vi "TDC_DAQV18_NewStructure.vi"(8 "error in (no error)":errorcluster, 9 "stop":bool, 10 "save data":bool, 11 "SMA mode":bool=TRUE) -> (3 "rate":dbl)   [LabVIEW 2017]
uses:
  <vilib>/Utility/file.llb/Write Delimited Spreadsheet (DBL).vi
  <vilib>/Utility/file.llb/Write Delimited Spreadsheet (I64).vi
panel:
  out "substring":string
  in  "factor":i32=128
  in  "displayCR":bool=TRUE
  in  "Counter Setting":dbl=100000.0 format="%#_13g"
  in  "replace dat":bool
  in  "append csv":bool=TRUE
  out "concatenated string":string
  out "number":u32=22
  out "element":string
  out "fine":u64=838 format="%x"
  in  "UDP Config":bool=TRUE
  in  "data  path":path=path "G:/tdc/2017"
  out "Array 6":u64[](array[numeric])
  out "cal 2":u64[](graph)
  in  "Thresholds (mV)":u16[](array[numeric])=[580, 580, 580, 580, 600, 600, 600, 600, 580, 580, 600, 600, 600, 600, 600, 600, 580, 580, 600, 600, 600, 600, 600, 600, 580, 580, 600, 600, 600, 600, 600, 600]
  out "error out 2":errorcluster={"status"=TRUE, "code"=1122, "source"="Dequeue Element in TDC_DAQV18_NewStructure.vi"}
  in  "display":bool=TRUE
  in  "Thresholds":u16=580
  in  "one key for threshold":bool=TRUE
  in  "RST":bool
  in  "通道数量":i32=64
  out "Cal Table":u32[](array[numeric])=[28636, 28570, 28472, 28284, 28524, 28354, 28408, 28049, 28174, 28071, 28126, 28086, 28151, 27908, 28025, 27898, 28233, 27859, 27914, 27888, 28140, 28038, 27911, 27738, 28022, 27827, 27982, 27675, 27862, 27768, 27841, 27799, 27874, 27627, 27754, 27650, 27959, 27594, 27633, 27606, 27668, 27555, 27455, 27220, 27394, 27187, 27334, 27119, 27301, 27220, 27267, 27235, 27336, 27057, 27150, 27031, 27376, 27049, 27063, 27028, 27283, 27180, 27100, 26881]
  in  "channel for cal":i32=62
  out "single":u32 format="%08x"
  out "channel number":u64
  in  "bytes to read":i32=320
  out "Calibration Counter":i32
  out "Event index":i32=97959
  out "cal":u32[](graph)=[0, 0, 0, 0, 0, 0, 0, 0, 0, 0, 0, 0, 0, 0, 0, 0, 0, 0, 0, 0, 0, 0, 0, 0, 0, 0, 0, 0, 0, 0, 0, 0, 0, 0, 0, 0, 0, 0, 0, 0, 0, 0, 0, 0, 0, 0, 0, 0, 0, 0, 0, 0, 0, 0, 0, 0, 0, 0, 0, 0, 0, 0, 0, 0, 0, 0, 0, 0, 0, 0, 0, 0, 0, 0, 0, 0, 0, 0, 0, 0, 0, 0, 0, 0, 0, 0, 0, 0, 0, 0, 0, 0, 0, 0, 0, 0, 0, 0, 0, 0, 0, 0, 0, 0, 0, 0, 0, 0, 0, 0, 0, 0, 0, 0, 0, 0, 0, 0, 0, 0, 0, 0, 0, 0, 0, 0, 0, 0, 0, 0, 0, 0, 0, 0, 0, 0, 0, 0, 0, 0, 0, 0, 0, 0, 0, 0, 0, 0, 0, 0, 0, 0, 0, 0, 0, 0, 0, 0, 0, 0, 0, 0, 0, 0, 0, 0, 0, 0, 0, 0, 0, 0, 0, 0, 0, 0, 0, 0, 0, 0, 0, 0, 0, 0, 0, 0, 0, 0, 0, 0, 0, 0, 0, 2, 54, 54, 14, 13, 87, 147, 41, 25, 155, 114, 17, 77, 15, 71, 56, 118, 81, 90, 49, 14, 113, 39, 20, 90, 64, 40, 165, 17, 96, 16, 10, 135, 156, 24, 21, 77, 15, 113, 60, 111, 60, 69, 56, 39, 25, 108, 23, 52, 40, 66, 77, 46, 18, 23, 25, 33, 46, 79, 55, 12, 43, 34, 54, 48, 32, 34, 28, 55, 22, 24, 21, 53, 50, 21, 11, 31, 77, 14, 70, 43, 17, 109, 25, 16, 16, 72, 32, 104, 58, 108, 13, 16, 11, 11, 72, 30, 49, 18, 45, 40, 66, 33, 22, 22, 74, 43, 18, 19, 21, 18, 60, 21, 31, 36, 29, 73, 97, 22, 11, 30, 9, 25, 193, 74, 57, 86, 69, 47, 59, 36, 30, 55, 41, 124, 44, 61, 22, 51, 50, 35, 27, 9, 64, 119, 23, 14, 164, 36, 42, 32, 43, 99, 31, 18, 26, 30, 31, 21, 113, 89, 30, 55, 19, 10, 21, 14, 46, 24, 51, 85, 44, 39, 50, 18, 26, 39, 30, 24, 32, 123, 21, 19, 90, 37, 44, 34, 33, 23, 68, 17, 29, 31, 65, 19, 61, 39, 31, 43, 29, 22, 10, 14, 11, 25, 86, 14, 22, 108, 89, 17, 47, 23, 15, 19, 146, 20, 31, 22, 74, 13, 22, 13, 120, 64, 70, 46, 27, 22, 133, 24, 44, 24, 20, 26, 110, 48, 68, 61, 65, 29, 49, 61, 92, 31, 33, 41, 54, 35, 24, 128, 22, 63, 41, 18, 84, 14, 25, 169, 23, 43, 15, 24, 172, 35, 124, 19, 31, 9, 11, 32, 134, 43, 65, 39, 44, 43, 34, 29, 13, 15, 74, 64, 26, 62, 44, 22, 21, 12, 14, 63, 43, 46, 39, 79, 28, 18, 24, 26, 73, 18, 22, 20, 21, 21, 45, 57, 75, 13, 62, 24, 20, 15, 60, 59, 77, 31, 32, 101, 20, 15, 29, 57, 76, 24, 48, 14, 20, 52, 70, 46, 31, 50, 8, 33, 45, 69, 28, 19, 14, 34, 17, 20, 68, 48, 88, 65, 48, 62, 27, 17, 28, 31, 70, 94, 13, 86, 14, 11, 31, 25, 51, 70, 22, 47, 24, 38, 30, 7, 11, 22, 25, 41, 15, 36, 52, 72, 54, 27, 28, 76, 34, 223, 31, 29, 41, 34, 92, 122, 60, 26, 43, 22, 56, 11, 24, 41, 50, 55, 18, 67, 41, 16, 30, 55, 27, 19, 61, 33, 85, 80, 79, 46, 14, 91, 48, 205, 23, 26, 18, 31, 58, 81, 35, 82, 83, 21, 37, 25, 26, 84, 60, 84, 13, 86, 69, 63, 74, 18, 117, 49, 45, 144, 12, 45, 13, 13, 74, 48, 19, 27, 51, 34, 25, 11, 11, 17, 100, 16, 10, 10, 59, 35, 84, 24, 26, 22, 20, 21, 11, 121, 83, 35, 36, 135, 15, 24, 41, 23, 27, 15, 35, 93, 35, 80, 24, 36, 29, 18, 16, 27, 17, 58, 12, 23, 32, 55, 89, 67, 14, 19, 26, 20, 122, 72, 55, 67, 25, 32, 18, 21, 46, 102, 133, 24, 22, 15, 47, 28, 29, 16, 17, 21, 26, 69, 27, 65, 58, 23, 21, 51, 56, 33, 62, 116, 37, 78, 49, 52, 75, 18, 48, 48, 16, 74, 24, 30, 58, 18, 32, 53, 19, 13, 9, 27, 13, 20, 38, 86, 118, 15, 12, 22, 31, 91, 25, 46, 133, 27, 15, 36, 45, 53, 133, 56, 18, 58, 16, 40, 46, 21, 88, 17, 25, 33, 41, 33, 7, 3, 20, 32, 12, 6, 15, 3, 20, 6, 3, 8, 6, 1, 3, 2, 2, 2, 0, 0, 0, 0, 0, 0, 0, 0, 0, 0, 0, 0, 0, 0, 0, 0, 0, 0, 0, 0, 0, 0, 0, 0, 0, 0, 0, 0, 0, 0, 0, 0, 0, 0, 0, 0, 0, 0, 0, 0, 0, 0, 0, 0, 0, 0, 0, 0, 0, 0, 0, 0, 0, 0, 0, 0, 0, 0, 0, 0, 0, 0, 0, 0, 0, 0, 0, 0, 0, 0, 0, 0, 0, 0, 0, 0, 0, 0, 0, 0, 0, 0, 0, 0, 0, 0, 0, 0, 0, 0, 0, 0, 0, 0, 0, 0, 0, 0, 0, 0, 0, 0, 0, 0, 0, 0, 0, 0, 0, 0, 0, 0, 0, 0, 0, 0, 0, 0, 0, 0, 0, 0, 0, 0, 0, 0, 0, 0, 0, 0, 0, 0, 0, 0, 0, 0, 0, 0, 0, 0, 0, 0, 0, 0, 0, 0, 0, 0, 0, 0, 0, 0, 0, 0, 0, 0, 0, 0, 0, 0, 0, 0, 0, 0, 0, 0, 0, 0, 0, 0, 0, 0, 0, 0, 0, 0, 0, 0, 0, 0, 0, 0, 0, 0, 0, 0, 0, 0, 0, 0, 0, 0, 0, 0, 0, 0, 0, 0, 0, 0, 0, 0, 0, 0, 0, 0, 0, 0, 0, 0, 0, 0, 0, 0, 0, 0, 0, 0, 0, 0, 0, 0, 0, 0, 0, 0, 0, 0, 0, 0, 0, 0, 0, 0, 0, 0, 0, 0, 0, 0, 0, 0, 0, 0, 0, 0, 0, 0, 0, 0, 0, 0, 0, 0, 0, 0, 0, 0, 0, 0, 0, 0, 0, 0, 0, 0, 0, 0, 0, 0, 0, 0, 0, 0, 0, 0, 0, 0, 0, 0, 0, 0, 0, 0, 0, 0, 0, 0, 0, 0, 0, 0, 0, 0, 0, 0, 0, 0, 0, 0, 0, 0, 0, 0, 0, 0, 0, 0, 0, 0, 0, 0, 0, 0, 0, 0, 0, 0, 0, 0, 0, 0, 0, 0, 0, 0, 0, 0, 0, 0, 0, 0, 0, 0, 0, 0, 0, 0, 0, 0, 0, 0, 0, 0, 0, 0, 0, 0, 0, 0, 0, 0, 0, 0, 0, 0, 0, 0, 0, 0, 0, 0, 0, 0, 0, 0, 0, 0, 0, 0, 0, 0, 0, 0, 0, 0, 0, 0, 0, 0, 0, 0, 0, 0, 0, 0, 0, 0, 0, 0, 0, 0, 0, 0, 0, 0, 0, 0, 0, 0, 0, 0, 0, 0, 0, 0, 0, 0, 0, 0, 0, 0, 0, 0, 0, 0, 0, 0, 0, 0, 0, 0, 0, 0, 0, 0, 0, 0, 0, 0, 0, 0, 0, 0, 0, 0, 0, 0, 0, 0, 0, 0, 0, 0, 0, 0, 0, 0, 0, 0, 0, 0, 0, 0, 0, 0, 0, 0, 0, 0, 0, 0, 0, 0, 0, 0, 0, 0, 0, 0, 0, 0, 0, 0, 0, 0, 0, 0, 0, 0, 0, 0, 0, 0, 0, 0, 0, 0, 0, 0, 0, 0, 0, 0, 0, 0, 0, 0, 0, 0, 0, 0, 0, 0, 0, 0, 0, 0, 0, 0, 0, 0, 0, 0, 0, 0, 0, 0, 0, 0, 0, 0, 0, 0, 0, 0, 0, 0, 0, 0, 0, 0, 0, 0, 0, 0, 0, 0, 0, 0, 0, 0, 0, 0, 0, 0, 0, 0, 0, 0, 0, 0, 0, 0, 0, 0, 0, 0, 0, 0, 0, 0, 0, 0, 0, 0, 0, 0, 0, 0, 0, 0, 0, 0, 0, 0, 0, 0, 0, 0, 0, 0, 0, 0, 0, 0, 0, 0, 0, 0, 0, 0, 0, 0, 0, 0, 0, 0, 0, 0, 0, 0, 0, 0, 0, 0, 0, 0, 0, 0, 0, 0, 0, 0, 0, 0, 0, 0, 0, 0, 0, 0, 0, 0, 0, 0, 0, 0, 0, 0, 0, 0, 0, 0, 0, 0, 0, 0, 0, 0, 0, 0, 0, 0, 0, 0, 0, 0, 0, 0, 0, 0, 0, 0, 0, 0, 0, 0, 0, 0, 0, 0, 0, 0, 0, 0, 0, 0, 0, 0, 0, 0, 0, 0, 0, 0, 0, 0, 0, 0, 0, 0, 0, 0, 0, 0, 0, 0, 0, 0, 0, 0, 0, 0, 0, 0, 0, 0, 0, 0, 0, 0, 0, 0, 0, 0, 0, 0, 0, 0, 0, 0, 0, 0, 0, 0, 0, 0, 0, 0, 0, 0, 0, 0, 0, 0, 0, 0, 0, 0, 0, 0, 0, 0, 0, 0, 0, 0, 0, 0, 0, 0, 0, 0, 0, 0, 0, 0, 0, 0, 0, 0, 0, 0, 0, 0, 0, 0, 0, 0, 0, 0, 0, 0, 0, 0, 0, 0, 0, 0, 0, 0, 0, 0, 0, 0, 0, 0, 0, 0, 0, 0, 0, 0, 0, 0, 0, 0, 0, 0, 0, 0, 0, 0, 0, 0, 0, 0, 0, 0, 0, 0, 0, 0, 0, 0, 0, 0, 0, 0, 0, 0, 0, 0, 0, 0, 0, 0, 0, 0, 0, 0, 0, 0, 0, 0, 0, 0, 0, 0, 0, 0, 0, 0, 0, 0, 0, 0, 0, 0, 0, 0, 0, 0, 0, 0, 0, 0, 0, 0, 0, 0, 0, 0, 0, 0, 0, 0, 0, 0, 0, 0, 0, 0, 0, 0, 0, 0, 0, 0, 0, 0, 0, 0, 0, 0, 0, 0, 0, 0, 0, 0, 0, 0, 0, 0, 0, 0, 0, 0, 0, 0, 0, 0, 0, 0, 0, 0, 0, 0, 0, 0, 0, 0, 0, 0, 0, 0, 0, 0, 0, 0, 0, 0, 0, 0, 0, 0, 0, 0, 0, 0, 0, 0, 0, 0, 0, 0, 0, 0, 0, 0, 0, 0, 0, 0, 0, 0, 0, 0, 0, 0, 0, 0, 0, 0, 0, 0, 0, 0, 0, 0, 0, 0, 0, 0, 0, 0, 0, 0, 0, 0, 0, 0, 0, 0, 0, 0, 0, 0, 0, 0, 0, 0, 0, 0, 0, 0, 0, 0, 0, 0, 0, 0, 0, 0, 0, 0, 0, 0, 0, 0, 0, 0, 0, 0, 0, 0, 0, 0, 0, 0, 0, 0, 0, 0, 0, 0, 0, 0, 0, 0, 0, 0, 0, 0, 0, 0, 0, 0, 0, 0, 0, 0, 0, 0, 0, 0, 0, 0, 0, 0, 0, 0, 0, 0, 0, 0, 0, 0, 0, 0, 0, 0, 0, 0, 0, 0, 0, 0, 0, 0, 0, 0, 0, 0, 0, 0, 0, 0, 0, 0, 0, 0, 0, 0, 0, 0, 0, 0, 0, 0, 0, 0, 0, 0, 0, 0, 0, 0, 0, 0, 0, 0, 0, 0, 0, 0, 0, 0, 0, 0, 0, 0, 0, 0, 0, 0, 0, 0, 0, 0, 0, 0, 0, 0, 0, 0, 0, 0, 0, 0, 0, 0, 0, 0, 0, 0, 0, 0, 0, 0, 0, 0, 0, 0, 0, 0, 0, 0, 0, 0, 0, 0, 0, 0, 0, 0, 0, 0, 0, 0, 0, 0, 0, 0, 0, 0, 0, 0, 0, 0, 0, 0, 0, 0, 0, 0, 0, 0, 0, 0, 0, 0, 0, 0, 0, 0, 0, 0, 0, 0, 0, 0, 0, 0, 0, 0, 0, 0, 0, 0, 0, 0, 0, 0, 0, 0, 0, 0, 0, 0, 0, 0, 0, 0, 0, 0, 0, 0, 0, 0, 0, 0, 0, 0, 0, 0, 0, 0, 0, 0, 0, 0, 0, 0, 0, 0, 0, 0, 0, 0, 0, 0, 0, 0, 0, 0, 0, 0, 0, 0, 0, 0, 0, 0, 0, 0, 0, 0, 0, 0, 0, 0, 0, 0, 0, 0, 0, 0]
  out "error out":errorcluster
  out "appended path":path=path "G:/tdc/2017/test_20250630_045315.dat"
  in  "filename":string="test"
  in  "Events":i32=110000 min=1
  in  "timeout (ms)":i32=10000
  in  "address":string="192.168.10.22"
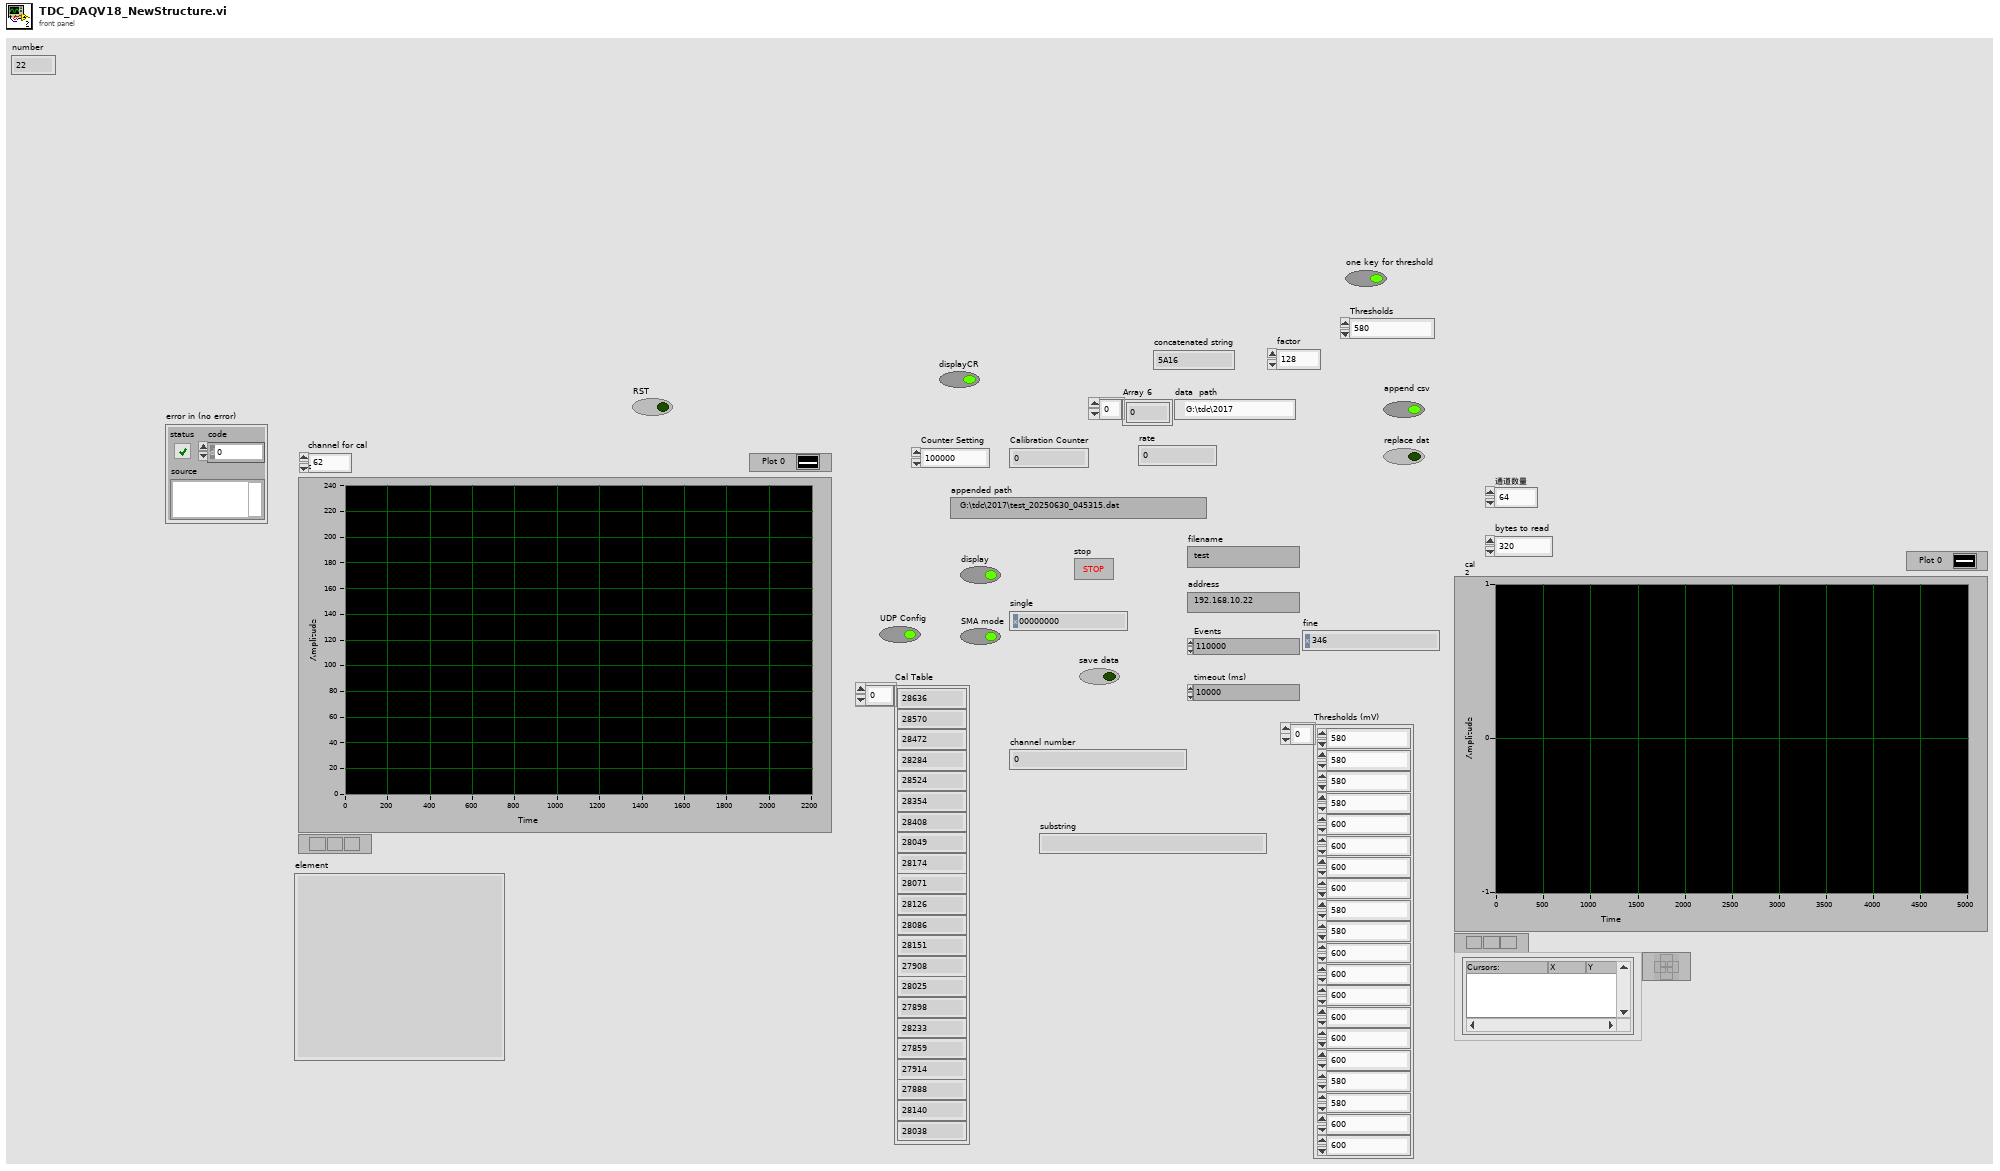
[diagram p1: front panel]
types:
  T1 = enum16{"open", "replace", "create", "open or create", "replace or create", "replace or create with confirmation"}
  T2 = enum16{"Standard", "Buffered", "CRLF", "Immediate"}
  T3 = enum16{"big-endian, network order", "native, host order", "little-endian"}
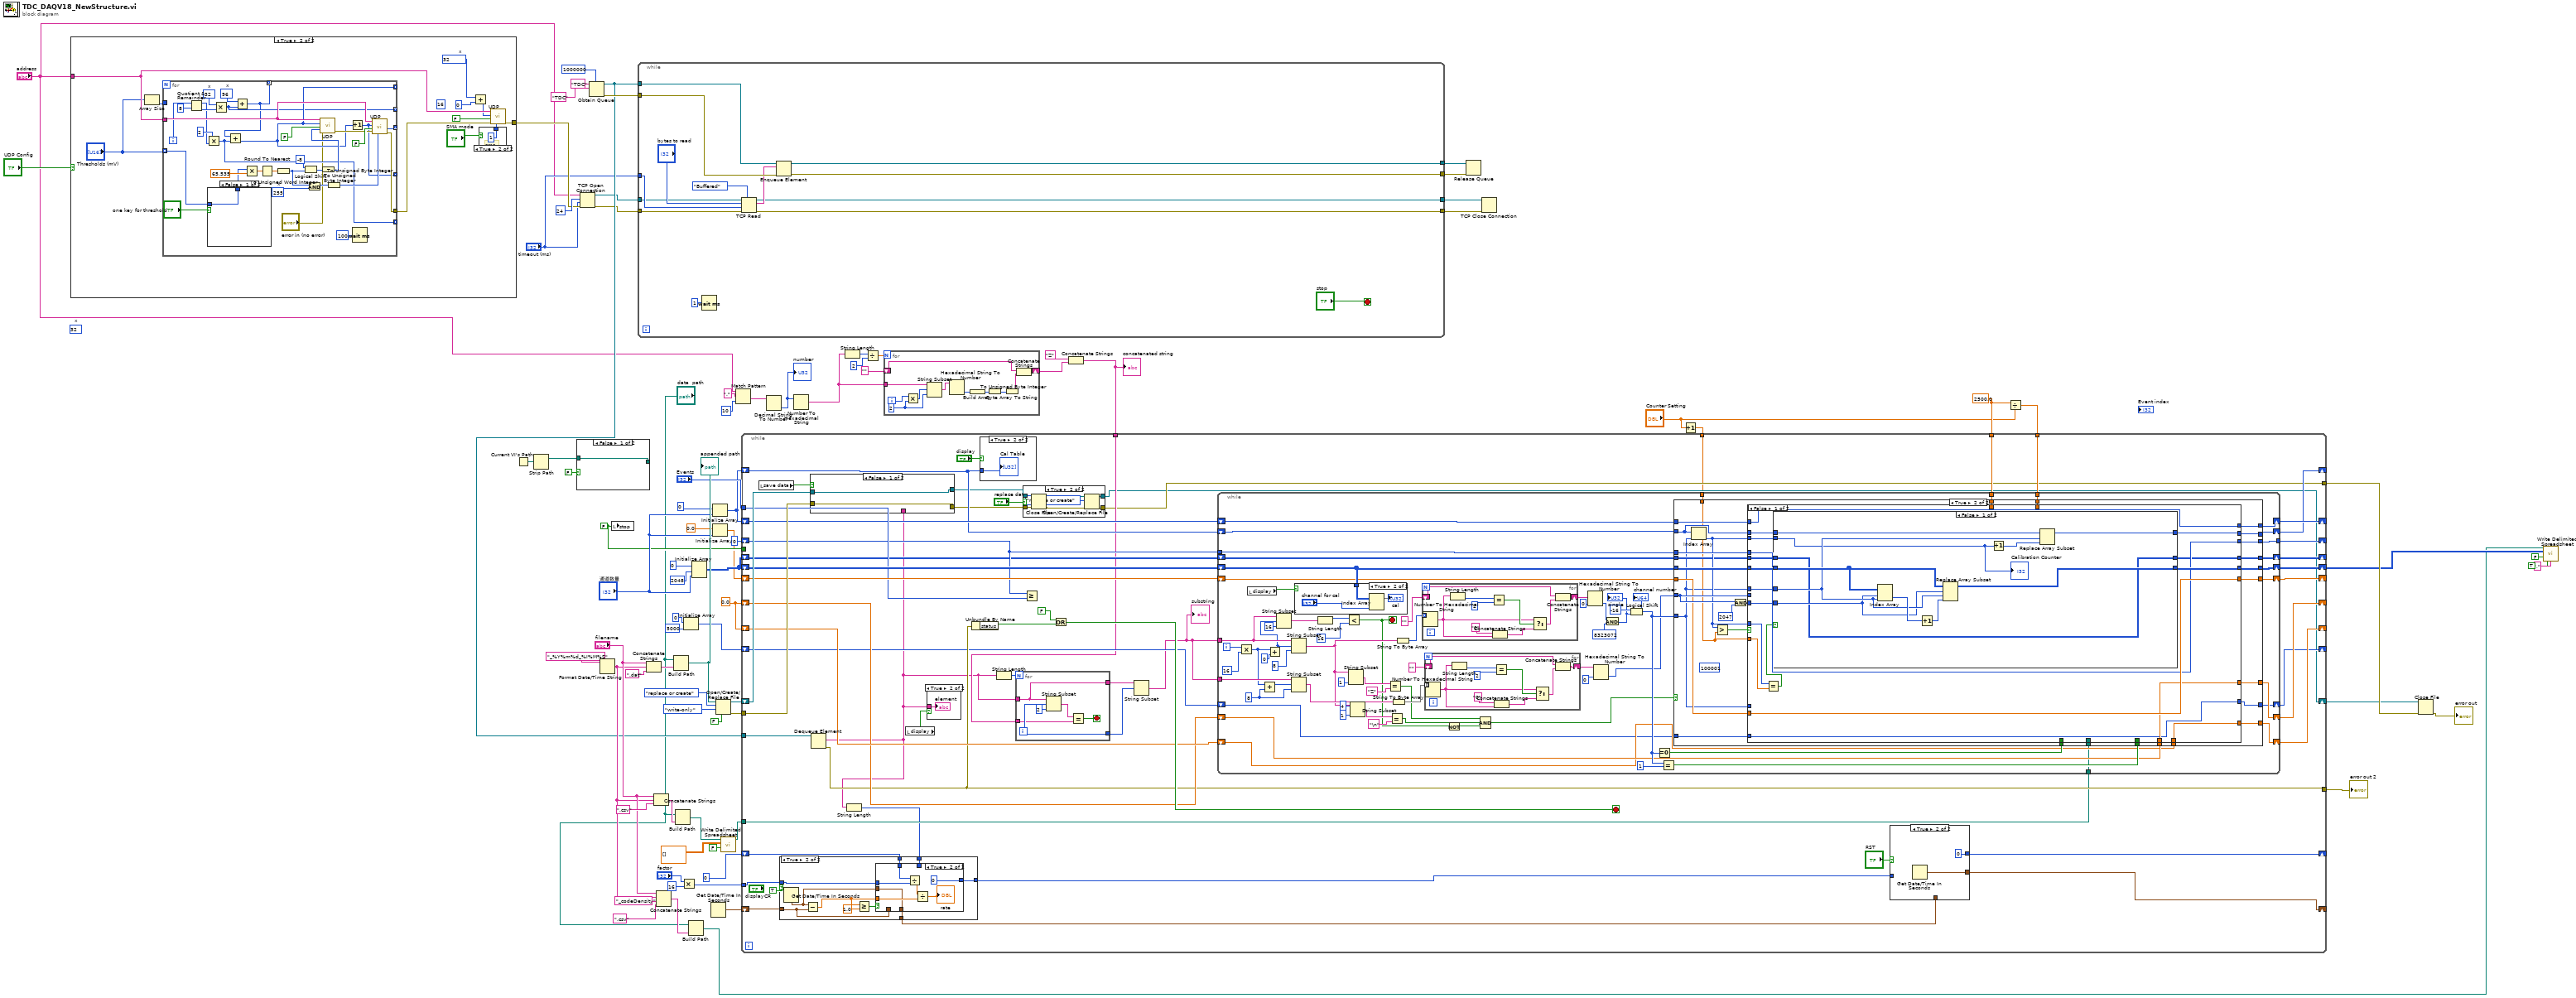
[diagram p0: block diagram]
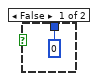
[diagram p3: hidden frame]
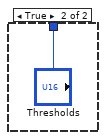
[diagram p4: hidden frame]
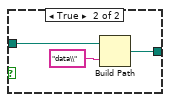
[diagram p5: hidden frame]
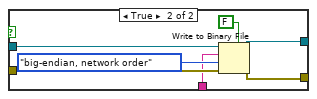
[diagram p7: hidden frame]
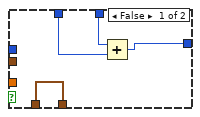
[diagram p10: hidden frame]
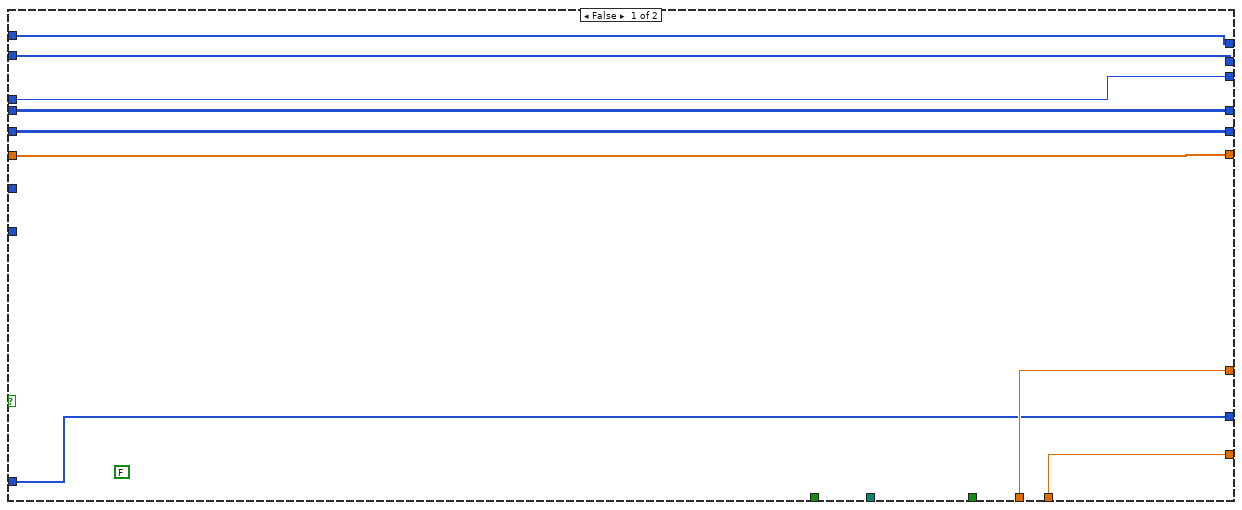
[diagram p14: hidden frame]
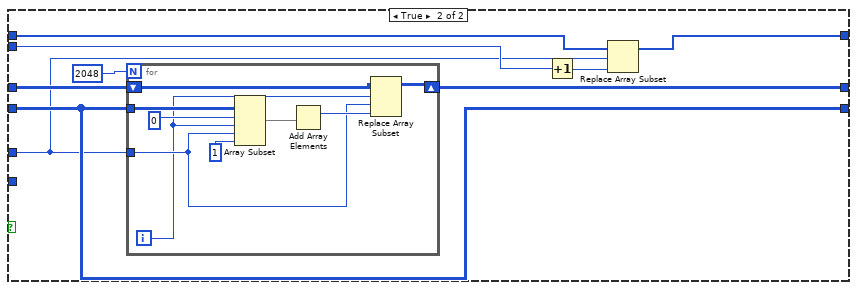
[diagram p15: hidden frame]
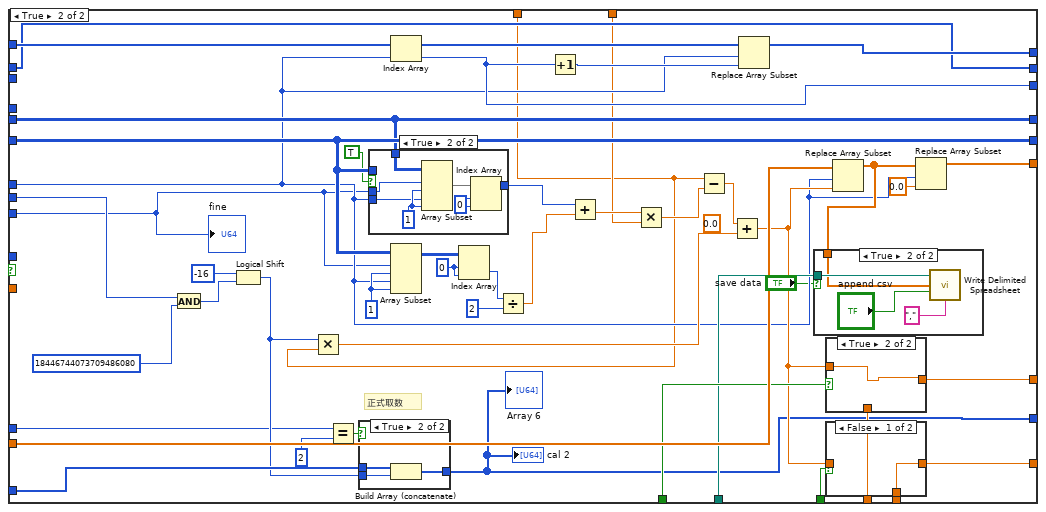
[diagram p16: hidden frame]
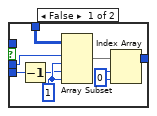
[diagram p19: hidden frame]
diagram:
  w9 = 2500.0 ("x")
  (unwired) u16 32  # x
  w53 = FALSE ("stop")
  w63 = 0.0
  n1 = case shown="True" "UDP Config" {
    tunnel: "address" -> [_ w96]
    tunnel: [_ w93] -> w54
    frame False {
    }
    frame True {
      (unwired) u32 16 ("Address")
      w87 = u16 32  # x
      n2 = Array Size(array="Thresholds (mV)") -> (size(s)=w90:i32)
      n3 = for {
        tunnel: w96 -> [w126]
        tunnel: "Thresholds (mV)" -> [w112] mode=indexing
        tunnel: [w120] -> _ mode=indexing
        tunnel: [w115] -> w94
        tunnel: w90 -> [_]
        tunnel: [w106] -> _ mode=indexing
        tunnel: [w105] -> _ mode=indexing
        tunnel: [w104] -> _ mode=indexing
        tunnel: [w103] -> _ mode=indexing
        tunnel: [w102] -> _ mode=indexing
        i -> [w107]
        w108 = u16 96  # x
        w109 = u16 32  # x
        w122 = u16 255  # x
        n4 = Quotient & Remainder(x=w107, y=8) -> (x-y*floor(x/y)=w101:i32, floor(x/y)=w110:i32)
        n5 = Multiply(x=2, y=w101) -> (x*y=w102:i32)
        n6 = case shown="False" "one key for threshold" {
          tunnel: [w132 "Thresholds"] -> w113
          tunnel: w112 -> [w132 _]
          frame False {
          }
          frame True {
          }
        }
        n7 = Multiply(x=w109, y=w110) -> (x*y=w104:i32)
        n8 = Add(x=w108, y=w104) -> (x+y=w103:i32)
        n9 = Add(x=w103, y=w102) -> (x+y=w106:i32)
        n10 = Multiply(x=w113, y=65.535) -> (x*y=w129:dbl)
        n11 = Round To Nearest(number=w129) -> (nearest integer value=w127:dbl)
        n12 = To Unsigned Word Integer(number=w127) -> (unsigned 16bit integer=w117:u16)
        n13 = Logical Shift(y=i16 -8, x=w117) -> (x << y=w124:u16)
        n14 = And(x=w117, y=w122) -> (x .and. y?=w121:u16)
        n15 = To Unsigned Byte Integer(number=w124) -> (unsigned 8bit integer=w123:u8)
        n16 = call "UDP.vi"("In"=w123, "error in (no error)"="error in (no error)", "Read (TRUE)"=FALSE, "Address"=w106, "IP address"=w126) -> ("error out"=w116:errorcluster)  [unwired: 3 in, 2 out]
        n17 = To Unsigned Byte Integer(number=w121) -> (unsigned 8bit integer=w119:u8)
        n18 = Increment(x=w106) -> (x+1=w105:i32)
        n19 = Wait (ms)(milliseconds to wait=u32 100) -> ()  [unwired: 1 out]
        n20 = call "UDP.vi"("In"=w119, "error in (no error)"=w116, "Read (TRUE)"=FALSE, "Address"=w105, "IP address"=w126) -> ("error out"=w115:errorcluster, "Out"=w120:u8)  [unwired: 3 in, 1 out]
      }
      n21 = Add(x=w87, y=u32 0 ("Address")) -> (x+y=w86:u32)
      n22 = case shown="True" "SMA mode" {
        tunnel: [u8 0 ("In") u8 1 ("In")] -> w92
        frame False {
        }
        frame True {
          # "sma"
        }
      }
      n23 = call "UDP.vi"("In"=w92, "error in (no error)"=w94, "Read (TRUE)"=FALSE, "Address"=w86, "IP address"=w96) -> ("error out"=w93:errorcluster)  [unwired: 3 in, 2 out]
    }
  }
  n24 = Current VI's Path() -> (path=w79:path)
  n25 = Strip Path(path=w79) -> (stripped path=w78:path)  [unwired: 1 out]
  n26 = case shown="False" FALSE {
    tunnel: w78 -> [w134 w136]
    tunnel: [w134 w135] -> _
    frame False {
    }
    frame True {
      n27 = Build Path(base path=w136, name or relative path="data\\") -> (appended path=w135:path)
    }
  }
  n28 = TCP Open Connection(address="address", remote port or service name=u16 24 ("port"), timeout ms (60000)="timeout (ms)", error in (no error)=w54) -> (connection ID=w37:refnum<k5>, error out=w38:errorcluster)  [unwired: 1 in]
  n29 = Obtain Queue(max queue size (-1, unlimited)=1000000, name (unnamed)="TDC", element data type="TDC" ("name (unnamed)")) -> (queue out=w39:refnum<queue>, error out=w40:errorcluster)  [unwired: 2 in, 1 out]
  n30 = Format Date/Time String(time format string (%c)="_%Y%m%d_%I%M%S") -> (date/time string=w51:string)  [unwired: 2 in]
  n31 = local write "stop"(w53) -> ()
  n32 = while {
    tunnel: w39 -> [w151]
    tunnel: w40 -> [w150]
    tunnel: w38 -> [w148]
    tunnel: "timeout (ms)" -> [w147]
    tunnel: w37 -> [w146]
    tunnel: [w144] -> w36
    tunnel: [w143] -> w35
    tunnel: [w141] -> w34
    tunnel: [w140] -> w33
    stop <- "stop" stop-if-true
    n33 = Wait (ms)(milliseconds to wait=u32 1) -> ()  [unwired: 1 out]
    n34 = TCP Read(connection ID=w146, bytes to read="bytes to read", error in (no error)=w148, 7:T2."Buffered" ("mode (standard)"), 9:w147) -> (connection ID out=w144:refnum<k5>, data out=w145:string, error out=w143:errorcluster)
    n35 = Enqueue Element(queue=w151, element=w145, error in (no error)=w150) -> (queue out=w141:refnum<queue>, error out=w140:errorcluster)  [unwired: 1 in, 1 out]
  }
  n36 = Concatenate Strings("filename", w51, ".dat") -> (w77:string)
  n37 = Concatenate Strings("filename", w51, ".csv") -> (w65:string)
  n38 = Concatenate Strings("filename", w51, "_codeDensity" ("string"), ".csv") -> (w48:string)
  n39 = Build Path(base path="data  path", name or relative path=w77) -> (appended path=w76:path)
  "appended path" <- w76
  n40 = Build Path(base path="data  path", name or relative path=w65) -> (appended path=w60:path)
  n41 = Multiply(x="factor", y=16) -> (x*y=w2:i32)
  n42 = Initialize Array(u32 0 ("element"), 5000 ("dimension size")) -> (w27:u32[])
  n43 = Build Path(base path="data  path", name or relative path=w48) -> (appended path=w45:path)
  n44 = Initialize Array(u32 0 ("element"), 2048 ("dimension size"), "通道数量") -> (w62:u32[][])
  n45 = Get Date/Time In Seconds() -> (seconds since 1Jan1904=w55:timestamp)
  n46 = Initialize Array(u32 0 ("element"), "通道数量") -> (w64:u32[])
  n47 = Initialize Array(0.0, "通道数量") -> (w29:dbl[])
  n48 = Open/Create/Replace File(file path (use dialog)=w76, operation (0:open)=T1."replace or create", access (0:read/write)=enum16{"read/write", "read-only", "write-only"}."write-only", disable buffering (F)=FALSE) -> (refnum out=w81:refnum<file>, error out=w80:errorcluster)  [unwired: 2 in, 1 out]
  n49 = call-poly <vilib>:"Write Delimited Spreadsheet.vi"("file path (dialog if empty)"=w60, "2D data"=dbl[][] [], "append to file? (new file:F)"=FALSE) -> ("new file path (Not A Path if cancelled)"=w59:path)  [unwired: 11 in, 1 out]
  n50 = Match Pattern(string="address", regular expression="." ("search string"), offset (0)=10) -> (after substring=w16:string)  [unwired: 3 out]
  n51 = Decimal String To Number(string=w16) -> (number=w15:i32)  [unwired: 2 in, 1 out]
  "number" <- w15
  n52 = Number To Hexadecimal String(2:w15) -> (0:w13:string)  [unwired: 1 in]
  n53 = String Length(string=w13) -> (length=w21:i32)
  n54 = Divide(x=w21, y=2) -> (x/y=w22:dbl)
  n55 = for {
    N: w22 -> [_]
    shift-right: [w162] -> w12
    shift-left: "" ("format string") -> [w161]
    tunnel: w13 -> [w152]
    i -> [w160]
    w154 = 2 ("y")
    n56 = Multiply(x=w160, y=w154) -> (x*y=w153:i32)
    n57 = String Subset(string=w152, offset (0)=w153, length (rest)=w154) -> (substring=w155:string)
    n58 = Hexadecimal String To Number(string=w155) -> (number=w159:u32)  [unwired: 2 in, 1 out]
    n59 = Build Array(w159) -> (w158:u32[])
    n60 = To Unsigned Byte Integer(number=w158) -> (unsigned 8bit integer=w157:u8[])
    n61 = Byte Array To String(unsigned byte array=w157) -> (string=w156:string)
    n62 = Concatenate Strings(w161, w156) -> (w162:string)
  }
  n63 = Concatenate Strings("Z", w12) -> (w11:string)
  "concatenated string" <- w11
  n64 = Release Queue(queue=w34, error in (no error)=w33) -> ()  [unwired: 1 in, 3 out]
  n65 = TCP Close Connection(connection ID=w36, error in (no error)=w35) -> ()  [unwired: 1 in, 2 out]
  n66 = Increment(x="Counter Setting") -> (x+1=w5:dbl)
  n67 = Divide(x=w9, y="Counter Setting") -> (x/y=w8:dbl)
  n68 = while {
    tunnel: w80 -> [w216]
    tunnel: [w190] -> w32
    tunnel: [w174] -> w73
    shift-right: [w213] -> w46
    shift-left: w62 -> [w214]
    shift-right: [w199] -> _
    shift-left: w29 -> [w212]
    tunnel: "Events" -> [w210]
    shift-right: [w209] -> _
    shift-left: w64 -> [w208]
    shift-right: [w207] -> _
    shift-left: u32 0 ("element") -> [w206]
    shift-right: [w205] -> _
    shift-left: w64 -> [w192]
    shift-right: [w204] -> _
    shift-left: w63 -> [w201]
    shift-right: [w203] -> _
    shift-left: w63 -> [w202]
    shift-right: [w194] -> _
    shift-left: w62 -> [w200]
    tunnel: w59 -> [w186]
    shift-right: [w198] -> _
    shift-left: 0 -> [w168]
    shift-right: [w196] -> _
    shift-left: w55 -> [w195]
    tunnel: w53 -> [_]
    tunnel: w39 -> [w191]
    shift-right: [w187] -> _
    shift-left: w27 -> [w188]
    tunnel: w11 -> [w182]
    tunnel: w9 -> [w180]
    tunnel: w8 -> [w179]
    shift-right: [w173] -> w7
    shift-left: w81 -> [w215]
    tunnel: w5 -> [w172]
    tunnel: w2 -> [w165]
    stop <- w211 stop-if-true
    n69 = local read "save data"() -> (w167:bool)
    n70 = Dequeue Element(queue=w191) -> (element=w178:string, error out=w190:errorcluster)  [unwired: 2 in, 2 out]
    n71 = case shown="False" w167 {
      tunnel: w216 -> [w218 w226]
      tunnel: w215 -> [w219 w225]
      tunnel: w178 -> [_ w222]
      tunnel: [w219 w221] -> w177
      tunnel: [w218 w220] -> w175
      frame False {
      }
      frame True {
        n72 = Write to Binary File(file (use dialog)=w225, data=w222, error in=w226, 5:FALSE ("prepend array or string size? (T)"), 9:T3."big-endian, network order" ("byte order (0:big-endian, network order)")) -> (refnum out=w221:refnum<file>, error out=w220:errorcluster)  [unwired: 1 in, 1 out]
      }
    }
    n73 = String Length(string=w178) -> (length=w169:i32)
    n74 = case shown="True" TRUE {
      tunnel: w195 -> [w243 w248]
      tunnel: [w243 w249] -> w171
      tunnel: w168 -> [w242 w247]
      tunnel: w169 -> [_ w246]
      tunnel: [w242 w245] -> w170
      tunnel: w165 -> [_ w244]
      frame False {
      }
      frame True {
        n75 = Get Date/Time In Seconds() -> (seconds since 1Jan1904=w250:timestamp)
        n76 = Subtract(x=w250, y=w248) -> (x-y=w252:dbl)
        n77 = Greater Or Equal?(x=w252, y=1.0) -> (x >= y?=w253:bool)
        n78 = case shown="True" w253 {
          tunnel: w252 -> [_ w264]
          tunnel: w250 -> [_ w262]
          tunnel: [w257 w262] -> w249
          tunnel: w248 -> [w257 _]
          tunnel: w247 -> [w256 w259]
          tunnel: w246 -> [w255 _]
          tunnel: [w254 0] -> w245
          tunnel: w244 -> [_ w258]
          frame False {
            n79 = Add(x=w255, y=w256) -> (x+y=w254:i32)
          }
          frame True {
            n80 = Divide(x=w259, y=w258) -> (x/y=w261:dbl)
            n81 = Divide(x=w261, y=w264) -> (x/y=→"rate":dbl)
          }
        }
      }
    }
    n82 = local read "display"() -> (w166:bool)
    n83 = case shown="True" w166 {
      tunnel: w178 -> [_ w217]
      frame False {
      }
      frame True {
        "element" <- w217
      }
    }
    n84 = Unbundle By Name(w190) -> ("status"=w189:bool)
    n85 = case shown="True" "display" {
      tunnel: w192 -> [_ w265]
      frame False {
      }
      frame True {
        "Cal Table" <- w265
      }
    }
    n86 = String Length(string=w178) -> (length=w185:i32)
    n87 = for {
      N: w185 -> [_]
      tunnel: w178 -> [w238]
      tunnel: [w238] -> w184
      tunnel: [w237] -> w183
      tunnel: w182 -> [w236]
      i -> [w237]
      stop <- w239 stop-if-true
      n88 = String Subset(string=w238, offset (0)=w237, length (rest)=2 ("length (rest)")) -> (substring=w240:string)
      n89 = Equal?(x=w240, y=w236) -> (x = y?=w239:bool)
    }
    n90 = case shown="True" "replace dat" {
      tunnel: w177 -> [w228 w234]
      tunnel: [w228 w233] -> w173
      tunnel: w175 -> [w227 w230]
      tunnel: [w227 w229] -> w174
      frame False {
      }
      frame True {
        n91 = Close File(refnum=w234, error in=w230) -> (path=w235:path, error out=w231:errorcluster)
        n92 = Open/Create/Replace File(file path (use dialog)=w235, error in=w231, operation (0:open)=T1."replace or create") -> (refnum out=w233:refnum<file>, error out=w229:errorcluster)  [unwired: 3 in, 1 out]
      }
    }
    n93 = Greater Or Equal?(x=w206, y=w210) -> ()  [unwired: 1 out]
    n94 = Or(x=FALSE, y=w189) -> (x .or. y?=w211:bool)
    n95 = String Subset(string=w184, offset (0)=w183) -> (substring=w163:string)  [unwired: 1 in]
    "substring" <- w163
    n96 = while {
      tunnel: w163 -> [w277]
      shift-right: [w333] -> w213
      shift-left: w214 -> [w331]
      shift-right: [w329] -> w199
      shift-left: w212 -> [w330]
      shift-right: [w324] -> w209
      shift-left: w208 -> [w323]
      tunnel: [w322] -> w207
      tunnel: w206 -> [w321]
      shift-right: [w319] -> w205
      shift-left: w192 -> [w320]
      shift-right: [w314] -> w204
      shift-left: w201 -> [w312]
      shift-right: [w310] -> w203
      shift-left: w202 -> [w311]
      tunnel: w186 -> [w309]
      shift-right: [w308] -> w194
      shift-left: w200 -> [w271]
      shift-right: [w305] -> w187
      shift-left: w188 -> [w306]
      tunnel: w163 -> [w297]
      tunnel: w180 -> [w279]
      tunnel: w179 -> [w278]
      tunnel: w172 -> [w270]
      i -> [w334]
      stop <- w273 stop-if-true
      w294 = 8 ("length (rest)")
      n97 = Multiply(x=w334, y=16 ("length (rest)")) -> (x*y=w295:i32)
      n98 = local read "display"() -> (w307:bool)
      n99 = Add(x=w295, y=w294) -> (x+y=w296:i32)
      n100 = Add(x=w295, y=0 ("length (rest)")) -> (x+y=w276:i32)
      n101 = String Subset(string=w277, offset (0)=w276, length (rest)=16 ("y")) -> (substring=w274:string)
      n102 = String Subset(string=w277, offset (0)=w276, length (rest)=8 ("length (rest)")) -> (substring=w280:string)
      n103 = String Subset(string=w297, offset (0)=w296, length (rest)=w294) -> (substring=w290:string)
      n104 = case shown="True" w307 {
        tunnel: w331 -> [_ w350]
        frame False {
        }
        frame True {
          n105 = Index Array(array=w350, index (col)="channel for cal") -> (element=→"cal":u32[])  [unwired: 1 in]
        }
      }
      n106 = String Length(string=w274) -> (length=w328:i32)
      n107 = Less?(x=w328, y=16) -> (x < y?=w273:bool)
      n108 = String Subset(string=w280, length (rest)=1 ("length (rest)")) -> (substring=w302:string)  [unwired: 1 in]
      n109 = String Subset(string=w280, offset (0)=4, length (rest)=1 ("length (rest)")) -> (substring=w281:string)
      n110 = Equal?(x=w302, y="Z" ("format string")) -> (x = y?=w283:bool)
      n111 = Equal?(x=w281, y="\n" ("format string")) -> (x = y?=w282:bool)
      n112 = String To Byte Array(string=w290) -> (unsigned byte array=w292:u8[])
      n113 = String To Byte Array(string=w280) -> (unsigned byte array=w336:u8[])
      n114 = for {
        shift-right: [w518] -> w288
        shift-left: "" ("format string") -> [w515]
        tunnel: w336 -> [w519] mode=indexing
        n115 = Number To Hexadecimal String(2:w519) -> (0:w511:string)  [unwired: 1 in]
        n116 = String Length(string=w511) -> (length=w517:i32)
        n117 = Equal?(x=w517, y=2) -> (x = y?=w514:bool)
        n118 = Concatenate Strings("0" ("format string"), w511) -> (w513:string)
        n119 = Select(t=w511, s=w514, f=w513) -> (s? t:f=w510:string)
        n120 = Concatenate Strings(w515, w510) -> (w518:string)
      }
      n121 = for {
        shift-right: [w346] -> w289
        shift-left: "" ("format string") -> [w338]
        tunnel: w292 -> [w347] mode=indexing
        n122 = Number To Hexadecimal String(2:w347) -> (0:w340:string)  [unwired: 1 in]
        n123 = String Length(string=w340) -> (length=w345:i32)
        n124 = Equal?(x=w345, y=2) -> (x = y?=w343:bool)
        n125 = Concatenate Strings("0" ("format string"), w340) -> (w342:string)
        n126 = Select(t=w340, s=w343, f=w342) -> (s? t:f=w339:string)
        n127 = Concatenate Strings(w338, w339) -> (w346:string)
      }
      n128 = Not(x=w273) -> (.not. x?=w272:bool)
      n129 = Compound Arithmetic op=AND(w283, w282, w272) -> (w300:bool)
      n130 = Hexadecimal String To Number(string=w288, default (0uL)=u64 0 ("default (0 U32)")) -> (number=w332:u64)  [unwired: 1 in, 1 out]
      n131 = Hexadecimal String To Number(string=w289, default (0uL)=u64 0 ("default (0 U32)")) -> (number=w287:u64)  [unwired: 1 in, 1 out]
      n132 = And(x=w332, y=u64 8323072 ("port")) -> (x .and. y?=w325:u64)
      "single" <- w325
      n133 = Logical Shift(y=i16 -16, x=w325) -> (x << y=w317:u64)
      "channel number" <- w317
      n134 = Equal To 0?(x=w317) -> (x = 0?=w315:bool)
      n135 = Equal?(x=w317, y=u64 1) -> (x = y?=w313:bool)
      n136 = case shown="True" w300 {
        tunnel: w287 -> [_ w389]
        tunnel: w321 -> [w356 w379]
        tunnel: w331 -> [w359 w388]
        tunnel: [w359 w387] -> w333
        tunnel: [w358 w384] -> w329
        tunnel: w330 -> [w358 w383]
        tunnel: w317 -> [_ w363]
        tunnel: w323 -> [w357 w382]
        tunnel: [w357 w381] -> w324
        tunnel: [w356 w380] -> w322
        tunnel: w320 -> [w355 w378]
        tunnel: [w355 w377] -> w319
        tunnel: w315 -> [_ w376]
        tunnel: w312 -> [w354 w375]
        tunnel: [w354 w374] -> w314
        tunnel: w313 -> [_ w373]
        tunnel: w311 -> [w353 w372]
        tunnel: [w353 w371] -> w310
        tunnel: w271 -> [w352 w369]
        tunnel: [w352 w368] -> w308
        tunnel: w309 -> [_ w367]
        tunnel: w306 -> [w351 w365]
        tunnel: [w351 w364] -> w305
        tunnel: w279 -> [_ w362]
        tunnel: w278 -> [_ w361]
        tunnel: w270 -> [_ w360]
        frame False {
          (unwired) FALSE
        }
        frame True {
          (unwired) 100001 ("y")
          n137 = Index Array(array=w378, index=w363) -> (element=w370:u32)
          n138 = Greater?(x=w370, y=w360) -> (0:w366:bool)
          n139 = And(x=w389, y=u64 2047 ("port")) -> (x .and. y?=w385:u64)
          n140 = case shown="False" w366 {
            tunnel: w389 -> [_ w482]
            tunnel: w388 -> [w407 w467]
            tunnel: [w406 w467] -> w387
            tunnel: w385 -> [w398 w440]
            tunnel: [w405 w451] -> w384
            tunnel: w383 -> [w405 w474]
            tunnel: w379 -> [w403 _]
            tunnel: w363 -> [w401 w449]
            tunnel: w382 -> [w404 w473]
            tunnel: [w404 w472] -> w381
            tunnel: [w403 w470] -> w380
            tunnel: w370 -> [w399 _]
            tunnel: w378 -> [w402 w469]
            tunnel: [w400 w469] -> w377
            tunnel: w376 -> [_ w462]
            tunnel: w375 -> [w397 w461]
            tunnel: [w397 w460] -> w374
            tunnel: w373 -> [_ w459]
            tunnel: w372 -> [w396 w458]
            tunnel: [w396 w457] -> w371
            tunnel: w370 -> [w394 _]
            tunnel: w360 -> [w391 _]
            tunnel: w369 -> [w393 w453]
            tunnel: [w392 w453] -> w368
            tunnel: w367 -> [_ w452]
            tunnel: w365 -> [w390 w446]
            tunnel: [w390 w444] -> w364
            tunnel: w363 -> [_ w441]
            tunnel: w362 -> [_ w438]
            tunnel: w361 -> [_ w439]
            frame False {
              n141 = Equal?(x=w394, y=w391) -> (x = y?=w395:bool)
              n142 = case shown="False" w395 {
                tunnel: w407 -> [w418 w424]
                tunnel: [w416 w424] -> w406
                tunnel: w402 -> [w414 w422]
                tunnel: w401 -> [w413 w419]
                tunnel: [w411 w421] -> w400
                tunnel: w399 -> [w410 w420]
                tunnel: w398 -> [w409 _]
                tunnel: w393 -> [w408 w426]
                tunnel: [w408 w425] -> w392
                frame False {
                  n143 = Index Array(array=w418, index (row)=w409, index (col)=w413) -> (element=w417:u32)
                  n144 = Increment(x=w417) -> (x+1=w415:u32)
                  n145 = Replace Array Subset(array=w418, new element=w415, index (row)=w409, index (col)=w413) -> (w416:u32[][])
                  n146 = Increment(x=w410) -> (x+1=w412:u32)
                  n147 = Replace Array Subset(array=w414, new element=w412, index=w413) -> (w411:u32[])
                  "Calibration Counter" <- w410
                }
                frame True {
                  n148 = for {
                    N: 2048 -> [_]
                    tunnel: w424 -> [w436]
                    tunnel: w419 -> [w429]
                    shift-right: [w431] -> w425
                    shift-left: w426 -> [w432]
                    i -> [w428]
                    n149 = Array Subset(array=w436, index (row)=0 ("索引"), length (row)=w428, index (col)=w429, length (col)=1 ("长度")) -> (w433:u32[][])
                    n150 = Add Array Elements(numeric array=w433) -> (sum=w430:u32)
                    n151 = Replace Array Subset(array=w432, new element=w430, index (row)=w428, index (col)=w429) -> (w431:u32[][])
                  }
                  n152 = Increment(x=w420) -> (x+1=w423:u32)
                  n153 = Replace Array Subset(array=w422, new element=w423, index=w419) -> (w421:u32[])
                }
              }
            }
            frame True {
              (unwired) 0.0 ("x")
              w464 = 0 ("索引 (行)")
              w466 = 1 ("长度")
              # "正式取数"
              n154 = And(x=w482, y=u64 18446744073709486080 ("port")) -> (x .and. y?=w479:u64)
              n155 = Logical Shift(y=i16 -16, x=w479) -> (x << y=w445:u64)
              n156 = Multiply(x=w445, y=w438) -> (x*y=w475:dbl)
              n157 = Equal?(x=w441, y=u32 2) -> (x = y?=w443:bool)
              n158 = case shown="True" w443 {
                tunnel: w446 -> [w483 w486]
                tunnel: w445 -> [_ w485]
                tunnel: [w483 w484] -> w444
                frame False {
                }
                frame True {
                  n159 = Build Array (concatenate)(w486, w485) -> (w484:u64[])
                }
              }
              "cal 2" <- w444
              "Array 6" <- w444
              n160 = case shown="True" TRUE {
                tunnel: [w493 w501] -> w477
                tunnel: w467 -> [_ _]
                tunnel: w449 -> [w498 w499]
                tunnel: w440 -> [w496 w504]
                tunnel: w453 -> [w497 w505]
                frame False {
                  w492 = 0 ("index (row)")
                  w495 = 1 ("长度")
                  n161 = Decrement(x=w498) -> (x-1=w491:u64)
                  n162 = Array Subset(array=w497, index (row)=w496, length (row)=w495, index (col)=w491, length (col)=w495) -> (w494:u32[][])
                  n163 = Index Array(array=w494, index (row)=w492, index (col)=w492) -> (element=w493:u32)
                }
                frame True {
                  w500 = 0 ("index (row)")
                  w503 = 1 ("长度")
                  n164 = Array Subset(array=w505, index (row)=w504, length (row)=w503, index (col)=w499, length (col)=w503) -> (w502:u32[][])
                  n165 = Index Array(array=w502, index (row)=w500, index (col)=w500) -> (element=w501:u32)
                }
              }
              n166 = Index Array(array=w473, index=w449) -> (element=w470:u32)
              n167 = Array Subset(array=w467, index (row)=w440, length (row)=w466, index (col)=w449, length (col)=w466) -> (w465:u32[][])
              n168 = Index Array(array=w465, index (row)=w464, index (col)=w464) -> (element=w463:u32)
              n169 = Divide(x=w463, y=u32 2) -> (x/y=w468:dbl)
              n170 = Increment(x=w470) -> (x+1=w471:u32)
              n171 = Add(x=w477, y=w468) -> (x+y=w476:dbl)
              n172 = Multiply(x=w476, y=w439) -> (x*y=w455:dbl)
              n173 = Subtract(x=w438, y=w455) -> (x-y=w437:dbl)
              n174 = Add(x=w437, y=w475) -> (x+y=w456:dbl)
              n175 = Replace Array Subset(array=w473, new element=w471, index=w449) -> (w472:u32[])
              n176 = case shown="True" w462 {
                tunnel: w456 -> [_ w509]
                tunnel: [w508 w509] -> w460
                tunnel: w461 -> [w508 _]
                frame False {
                }
                frame True {
                }
              }
              n177 = case shown="False" w459 {
                tunnel: [w506 w507] -> w457
                tunnel: w458 -> [w506 _]
                tunnel: w456 -> [_ w507]
                frame False {
                }
                frame True {
                }
              }
              n178 = Replace Array Subset(array=w474, new element=w456, index=w449) -> (w450:dbl[])
              n179 = case shown="True" "save data" {
                tunnel: w452 -> [_ w490]
                tunnel: w450 -> [_ w488]
                frame False {
                }
                frame True {
                  n180 = call-poly <vilib>:"Write Delimited Spreadsheet.vi"("file path (dialog if empty)"=w490, "1D data"=w488, "append to file? (new file:F)"="append csv", "delimiter (\\t)"="," ("delimiter (\\t)")) -> ()  [unwired: 10 in, 2 out]
                }
              }
              n181 = Replace Array Subset(array=w450, new element=0.0 ("new element/subarray"), index=w449) -> (w451:dbl[])
              "fine" <- w440
            }
          }
        }
      }
    }
    n182 = case shown="True" "RST" {
      tunnel: w170 -> [w267 _]
      tunnel: [w267 0] -> w198
      tunnel: [w266 w268] -> w196
      tunnel: w171 -> [w266 _]
      frame False {
      }
      frame True {
        n183 = Get Date/Time In Seconds() -> (seconds since 1Jan1904=w268:timestamp)
      }
    }
  }
  "error out 2" <- w32
  n184 = Close File(refnum=w7, error in=w73) -> (error out=→"error out":errorcluster)  [unwired: 1 out]
  n185 = call-poly <vilib>:"Write Delimited Spreadsheet.vi"("file path (dialog if empty)"=w45, "2D data"=w46, "append to file? (new file:F)"=FALSE, "transpose? (no:F)"=TRUE, "delimiter (\\t)"="," ("delimiter (\\t)")) -> ()  [unwired: 9 in, 2 out]
